vi "IngenieursAnsicht.vi"() -> (3 "Cluster":T1)   [LabVIEW 2018]
doc: "Das soll ein Frontpanel sein, welches einem die aktuellsten internen Parameter angibt wie zB. einen Temperaturverlaufsgraph."
panel:
  # "TODO: hier noch alle Anzeigen zum Cluster hinzufügen, welche für den Entwickler interessant wären zu sehen"
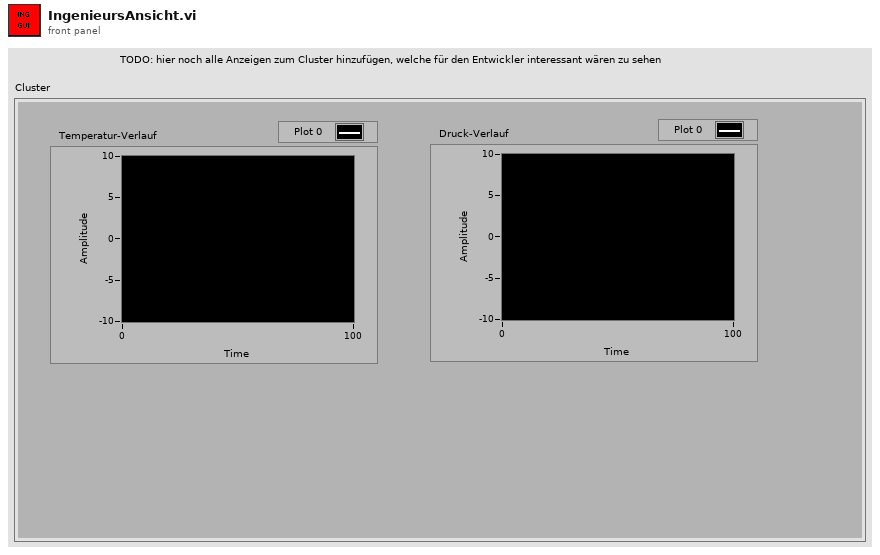
[diagram p1: front panel]
types:
  T1 = cluster{"Temperatur-Verlauf":dbl, "Druck-Verlauf":dbl}
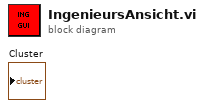
[diagram p0: block diagram]
diagram:
